vi "Boolean Toggle.vi"(1 "Input":bool) -> (21 "Output":bool)   [LabVIEW 2012]
doc: "Changes a standard boolean input to a toggled boolean output."
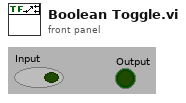
[diagram p1: front panel]
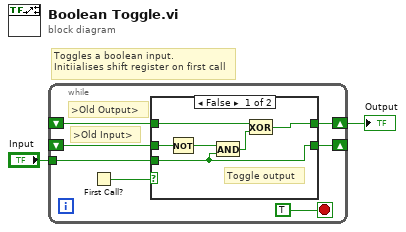
[diagram p0: block diagram]
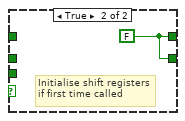
[diagram p2: hidden frame]
diagram:
  # "Toggles a boolean input.\nInitiialises shift register on first call"
  n1 = while {
    shift-right: [w9] -> w2
    shift-left: _ -> [w8]
    shift-right: [w4] -> _
    shift-left: _ -> [w6]
    tunnel: "Input" -> [w5]
    stop <- TRUE stop-if-true
    # ">Old Input>"
    # ">Old Output>"
    n2 = First Call?() -> (First Call?: T/F=w3:bool)
    n3 = case shown="False" w3 {
      tunnel: [w12 w16] -> w9
      tunnel: w8 -> [w10 _]
      tunnel: w6 -> [w13 _]
      tunnel: w5 -> [w14 _]
      tunnel: [w14 w16] -> w4
      frame False {
        # "Toggle output"
        n4 = Not(x=w13) -> (.not. x?=w15:bool)
        n5 = And(x=w15, y=w14) -> (x .and. y?=w11:bool)
        n6 = Exclusive Or(1:w11, 2:w10) -> (0:w12:bool)
      }
      frame True {
        w16 = FALSE
        # "Initialise shift registers\nif first time called"
      }
    }
  }
  "Output" <- w2
